vi "CameraVision_Demo_v02.vi"() -> (4 "图像时间戳":u32=16532020 format="%_32g")   [LabVIEW 2015]
uses:
  MVCAMSDK.dll
  <vilib>/Analysis/NI_AALBase.lvlib
panel:
  out "variance 2":dbl caption="方差2" format="%0.2f"
  out "光强图 2":u64[](graph)
  out "variance":dbl caption="方差" format="%0.2f"
  out "相机图像":T1(plugin-control)
  out "光强图":u64[](graph)
  in  "自定义分辨率设置":bool
  in  "ROI分辨率":T2
  in  "预设分辨率设置":bool
  in  "预设分辨率":T3(radio)
  out "帧速":u32
  out "帧间耗时\n单位：（0.1ms）":u32
  in  "相机枚举":T4(ring)
  in  "自动曝光模式":bool=TRUE caption="软触发"
  in  "手动曝光模式":bool caption="软触发"
  in  "曝光时间，单位微秒":dbl=11000.0 format="%#_6f"
  in  "硬触发模式":bool caption="软触发"
  in  "软触发模式":bool caption="软触发"
  in  "连续模式":bool caption="软触发"
  in  "软触发一帧":bool caption="软触发"
  in  "读取自定义数据":bool
  out "从相机中读出的字符串(32字节)":string
  in  "写入自定义数据":bool
  in  "要写入相机的字符串(32字节)":string
  in  "拍照":bool
  in  "相机参数":bool=TRUE
  in  "Stop":bool
  in  "激活预览":bool=TRUE
  out "Image":T1(plugin-control)
  # "写入自定义数据"
  # "相机原生分辨率设置"
  # "触发设置"
  # "曝光设置"
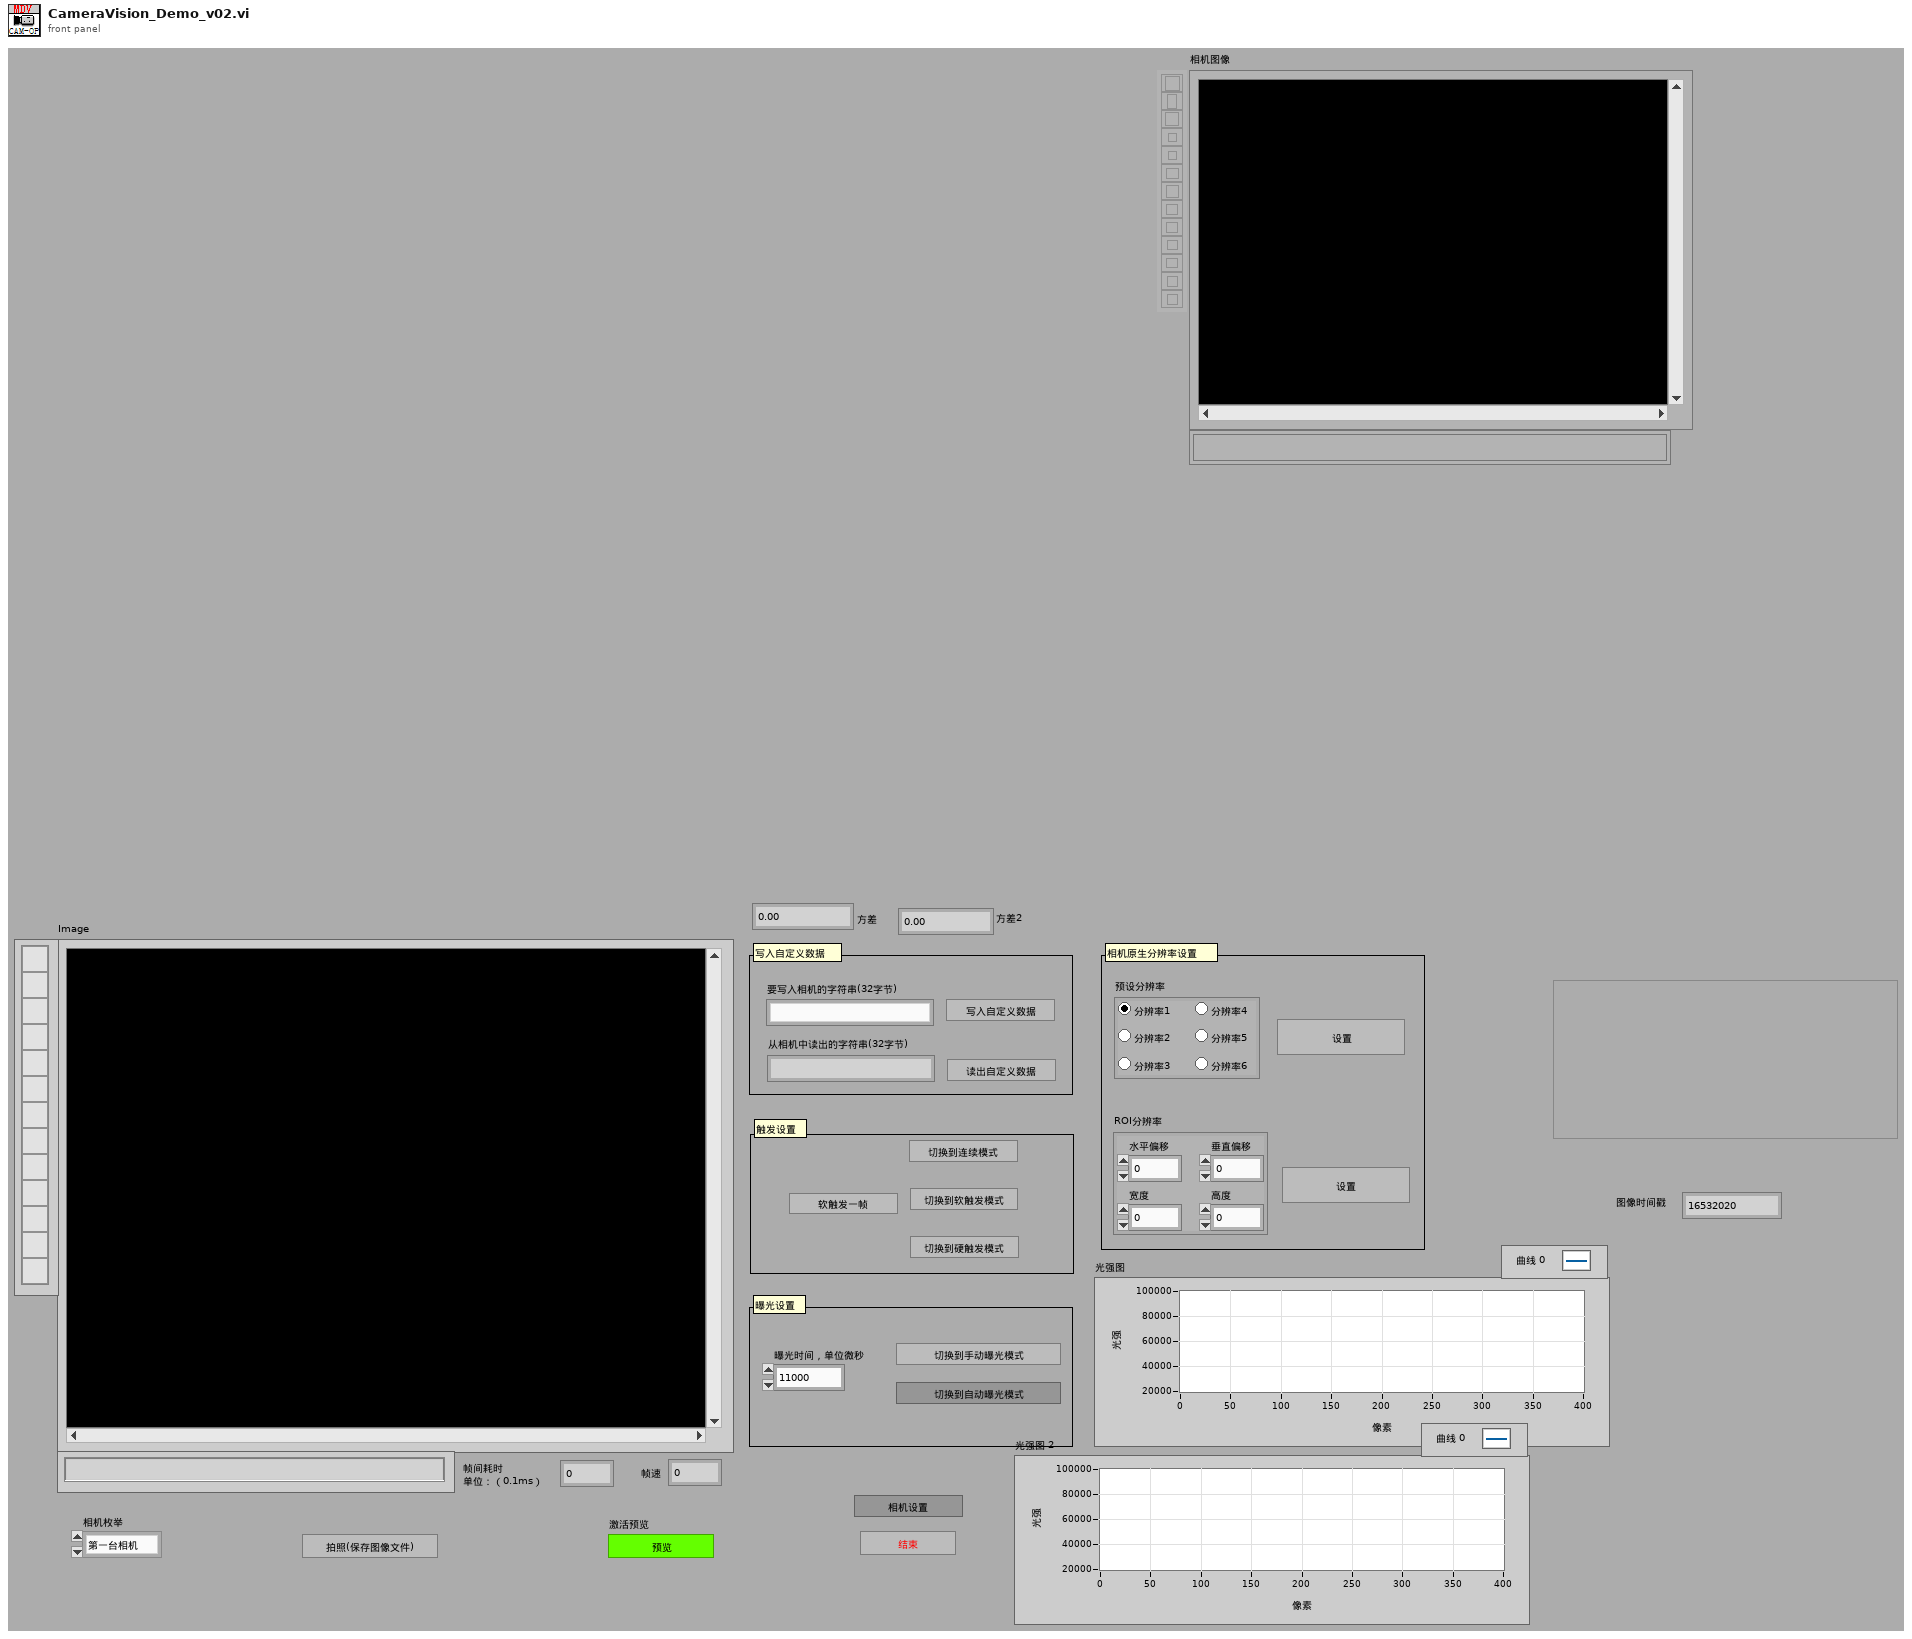
[diagram p1: front panel]
types:
  T1 = typedef "IMAQ Image.ctl" = refnum<image>
  T2 = cluster{"水平偏移":dbl, "垂直偏移":dbl, "宽度":dbl, "高度":dbl}
  T3 = enum32{"分辨率1", "分辨率2", "分辨率3", "分辨率4", "分辨率5", "分辨率6"}
  T4 = enum16{"第一台相机", "第二台相机", "第三台相机", "第四台相机", "第五台相机"}
  T5 = typedef "Image Type" = u32
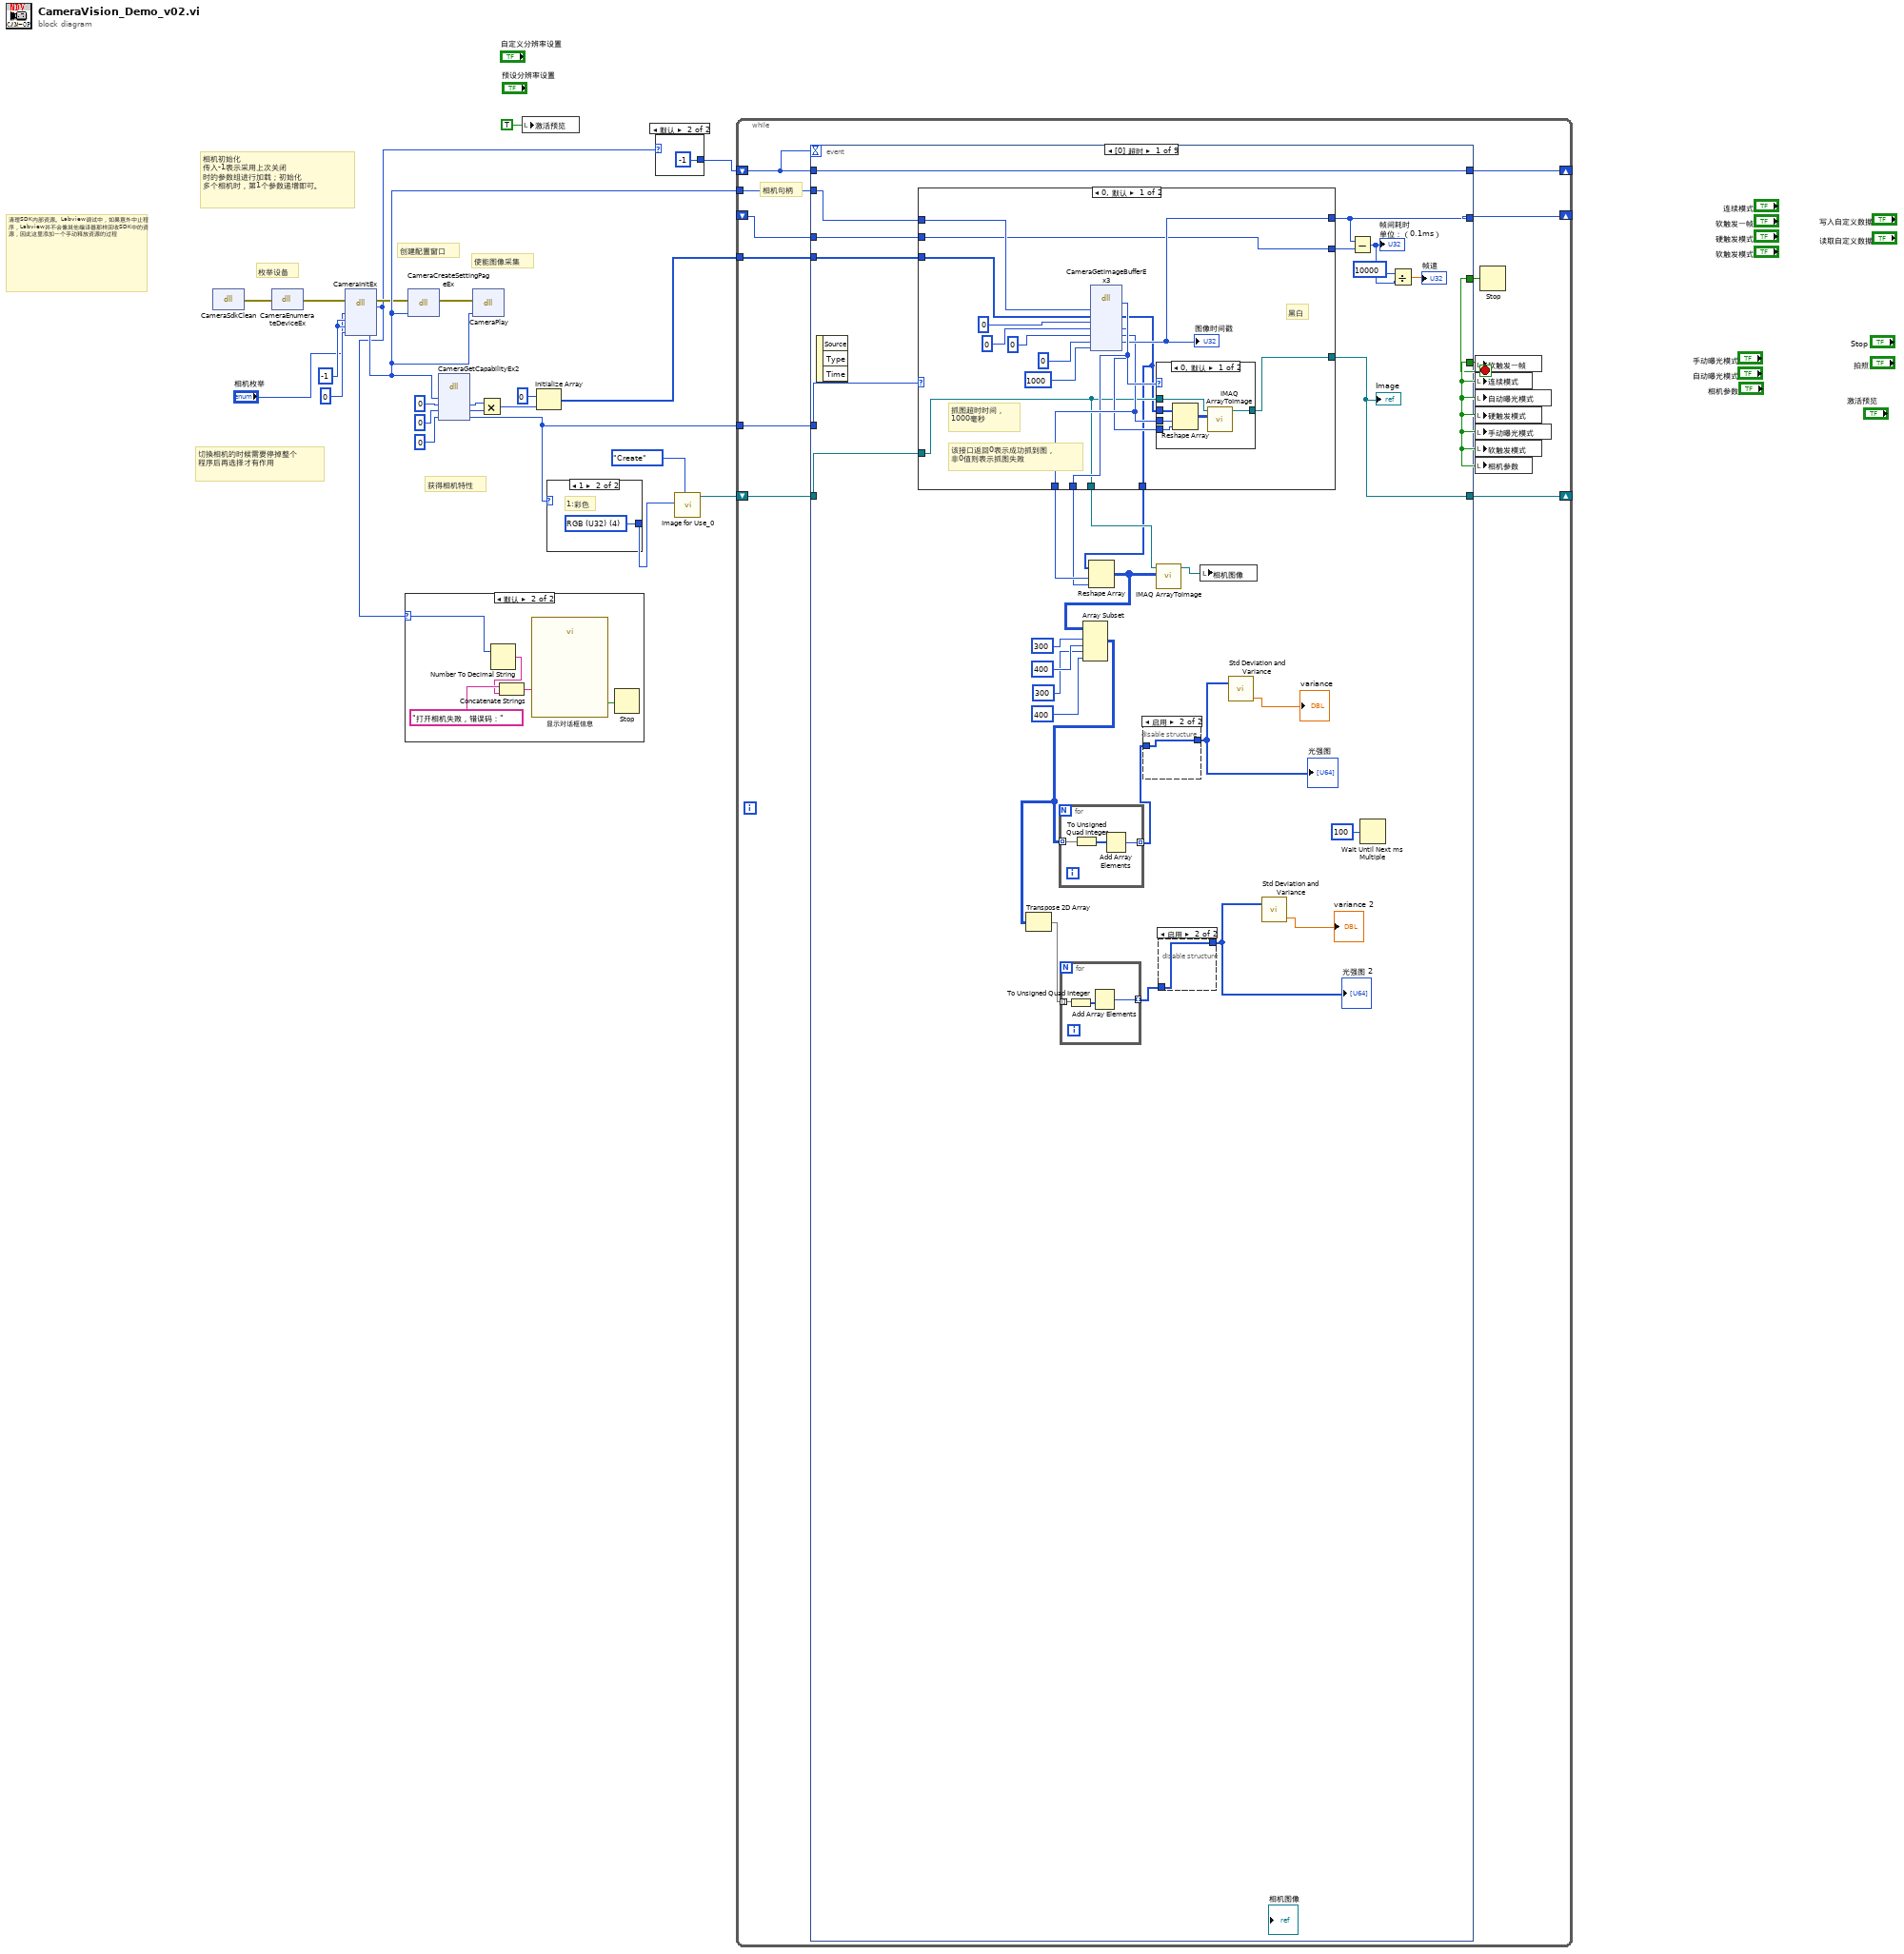
[diagram p0: block diagram]
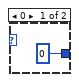
[diagram p2: hidden frame]
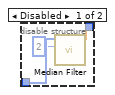
[diagram p4: hidden frame]
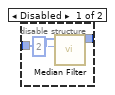
[diagram p5: hidden frame]
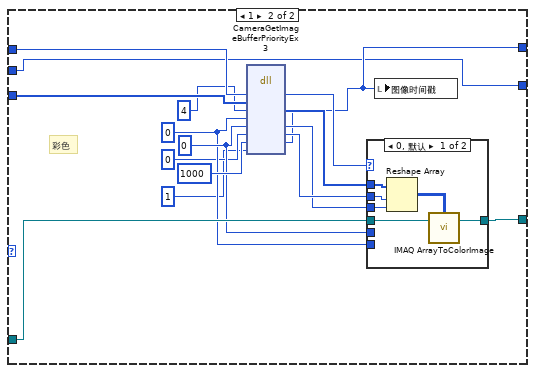
[diagram p7: hidden frame]
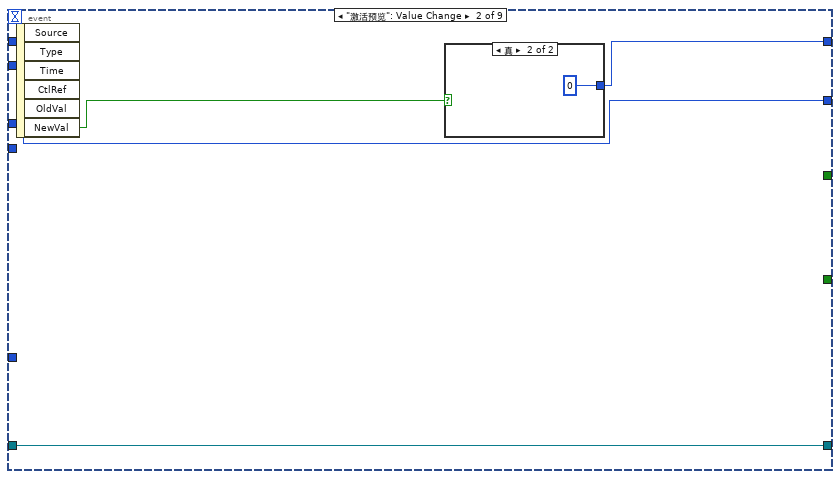
[diagram p9: hidden frame]
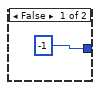
[diagram p10: hidden frame]
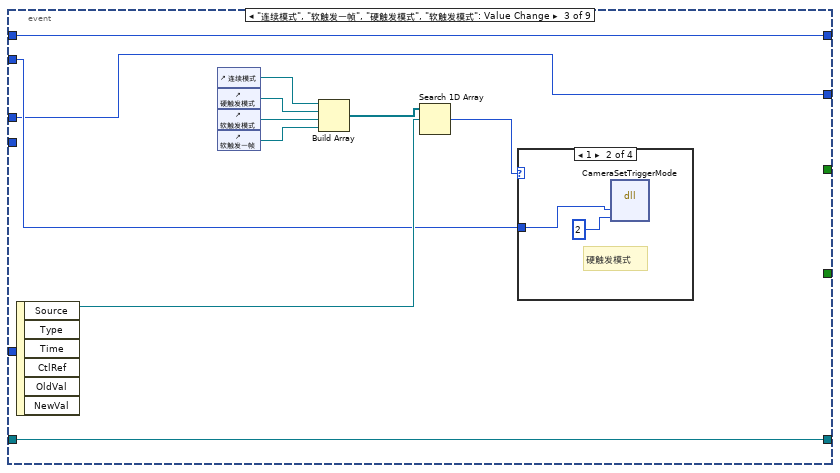
[diagram p11: hidden frame]
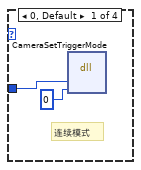
[diagram p12: hidden frame]
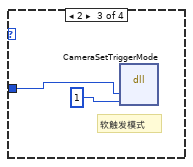
[diagram p13: hidden frame]
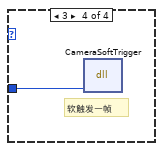
[diagram p14: hidden frame]
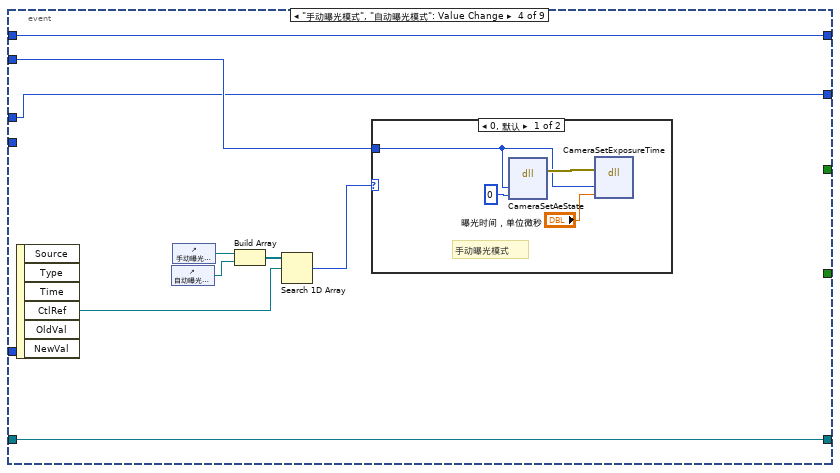
[diagram p15: hidden frame]
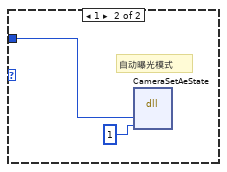
[diagram p16: hidden frame]
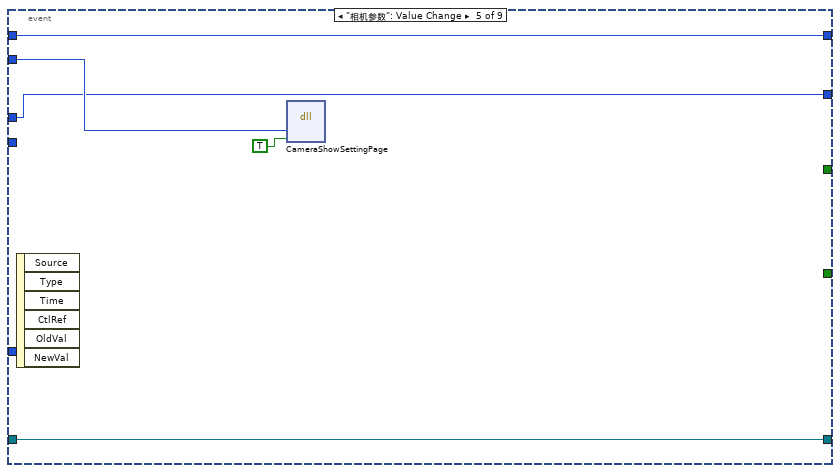
[diagram p17: hidden frame]
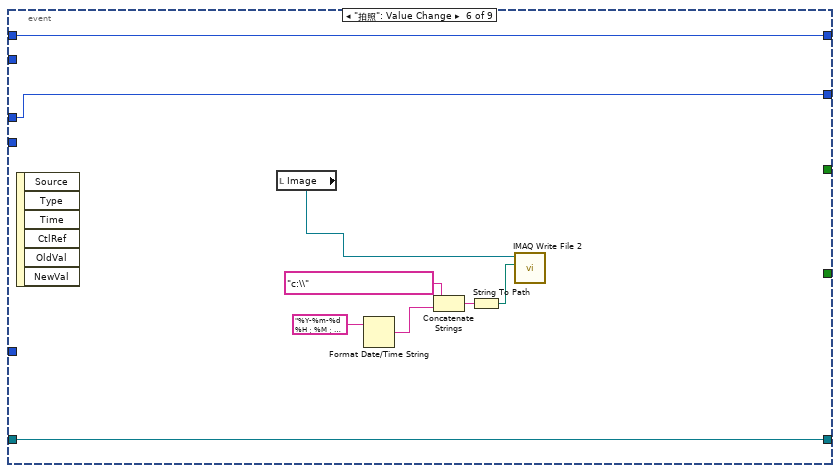
[diagram p18: hidden frame]
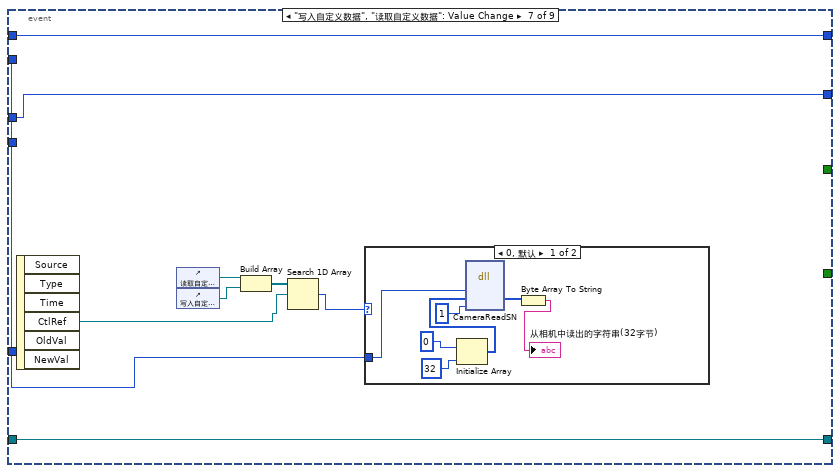
[diagram p19: hidden frame]
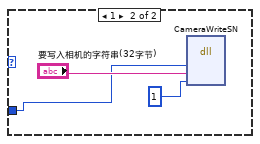
[diagram p20: hidden frame]
diagram:
  w20 = -1
  # "切换相机的时候需要停掉整个\n程序后再选择才有作用"
  # "清理SDK内部资源。Labview调试中，如果意外中止程序，Labview并不会像其他编译器那样回收SDK中的资源，因此这里添加一个手动释放资源的过程"
  # "使能图像采集"
  # "获得相机特性"
  # "创建配置窗口"
  # "相机初始化\n传入-1表示采用上次关闭\n时的参数组进行加载；初始化\n多个相机时，第1个参数递增即可。"
  # "枚举设备"
  n1 = dll-call lib="MVCAMSDK.dll" fn="CameraSdkClean"() -> (error out=w21:errorcluster)  [unwired: 4 in, 1 out]
  n2 = dll-call lib="MVCAMSDK.dll" fn="CameraEnumerateDeviceEx"(error in=w21) -> (error out=w18:errorcluster)  [unwired: 3 in, 1 out]
  n3 = dll-call lib="MVCAMSDK.dll" fn="CameraInitEx"(error in=w18, "相机索引值"="相机枚举", "参数加载方式"=w20, "要加载的参数组索引"=w20, "相机句柄"=0) -> (error out=w7:errorcluster, "返回类型"=w2:i32, "相机句柄"=w9:i32)  [unwired: 5 in, 1 out]
  n4 = case shown="默认" w2 {
    selector: w2 -> [_ w27]
    frame 0 {
    }
    frame Default {
      n5 = Number To Decimal String(number=w27) -> (decimal integer string=w24:string)  [unwired: 1 in]
      n6 = Concatenate Strings("打开相机失败，错误码：" ("字符串"), w24) -> (w26:string)
      n7 = call "显示对话框信息"("Message"=w26) -> ("结束"=w28:bool)  [unwired: 9 in, 1 out]
      n8 = Stop(stop? (T)=w28) -> ()
    }
  }
  n9 = dll-call lib="MVCAMSDK.dll" fn="CameraCreateSettingPageEx"(error in=w7, "相机句柄"=w9) -> (error out=w10:errorcluster)  [unwired: 4 in, 1 out]
  n10 = dll-call lib="MVCAMSDK.dll" fn="CameraGetCapabilityEx2"("相机句柄"=w9, "图像最大宽度"=0, "图像最大高度"=0, "是否是彩色相机(返回0:黑白;1:彩色)"=0) -> ("图像最大宽度"=w12:i32, "图像最大高度"=w11:i32, "是否是彩色相机(返回0:黑白;1:彩色)"=w6:i32)  [unwired: 5 in, 2 out]
  n11 = dll-call lib="MVCAMSDK.dll" fn="CameraPlay"(error in=w10, "相机句柄"=w9) -> ()  [unwired: 4 in, 2 out]
  n12 = Multiply(x=w12, y=w11) -> (x*y=w16:i32)
  n13 = local write "激活预览"(TRUE ("激活预览")) -> ()
  n14 = Initialize Array(0, w16) -> (w8:i32[])
  n15 = case shown="1" w6 {
    tunnel: [_ w29] -> w22
    frame 0, Default {
      # "0:黑白;"
    }
    frame 1 {
      w29 = T5 4 items=["Grayscale (U8)", "Grayscale (I16)", "Grayscale (SGL)", "Complex (CSG)", "RGB (U32)", "HSL (U32)", "RGB (U64)", "Grayscale (U16)"] ("Image Type")
      # "1:彩色"
    }
  }
  n16 = case shown="默认" w2 {
    tunnel: [0 -1] -> w1
    frame 0 {
    }
    frame Default {
    }
  }
  n17 = call "Image for Use_0.vi"("Command"=enum16{"Create", "Use", "Copy in", "Dispose"}."Create", "Image Type"=w22) -> ("Image out"=w5:T1)  [unwired: 8 in, 1 out]
  n18 = while {
    tunnel: w9 -> [w39]
    tunnel: w8 -> [w41]
    tunnel: w6 -> [w42]
    shift-right: [w38] -> _
    shift-left: w1 -> [w37]
    shift-right: [w35] -> _
    shift-left: w5 -> [w40]
    shift-right: [w34] -> _
    shift-left: _ -> [w33]
    stop <- w32 stop-if-true
    # "相机句柄"
    n19 = event shown="[0] 超时" {
      selector: _ -> [_ _ _ _ _ _ _ _ _]
      dyn-events: _ -> [_ _ _ _ _ _ _ _ _]
      timeout: w37 -> [_ _ _ _ _ _ _ _ _]
      tunnel: [_ _ _ _ _ _ _ _ TRUE] -> w32
      tunnel: w41 -> [w72 _ _ _ _ _ _ _ _]
      tunnel: w42 -> [w71 _ _ _ _ _ _ _ _]
      tunnel: w39 -> [w73 _ w141 w159 w174 _ w188 w211 w291]
      tunnel: w40 -> [w70 w134 w140 w158 w173 w178 w187 w213 w289]
      tunnel: [w69 w135 w142 w160 w175 w179 w189 w214 w292] -> w38
      tunnel: w37 -> [w69 _ w142 w160 w175 w179 w189 w214 w292]
      tunnel: [_ _ _ _ _ _ _ _ FALSE] -> w36
      tunnel: [w68 w134 w140 w158 w173 w178 w187 w213 w289] -> w35
      tunnel: [w65 w133 w139 w157 w172 w177 w186 w205 w288] -> w34
      tunnel: w33 -> [w67 w133 w139 w157 w172 w177 w186 w205 w288]
      event Timeout {
        n20 = event-data() -> ()  [unwired: 1 in, 3 out]
        n21 = case shown="0, 默认" w71 {
          tunnel: w72 -> [w102 w125]
          tunnel: w70 -> [w89 w124]
          tunnel: w73 -> [w94 w123]
          tunnel: [w95 w113] -> w68
          tunnel: [w93 w112] -> w65
          tunnel: w67 -> [w92 w111]
          tunnel: [w92 w111] -> w66
          tunnel: [w91 _] -> w59
          tunnel: [w90 _] -> w58
          tunnel: [w89 _] -> w57
          tunnel: [w88 _] -> w56
          frame 0, Default {
            # "黑白"
            # "该接口返回0表示成功抓到图，\n非0值则表示抓图失败"
            # "抓图超时时间，\n1000毫秒"
            n22 = dll-call lib="MVCAMSDK.dll" fn="CameraGetImageBufferEx3"("相机句柄"=w94, "图像数据缓冲区"=w102, "图像输出格式(0:8位灰度;1:24位彩色;2:32位彩色，3：BGR24彩色 4：BGRA32位彩色)"=0, "图像宽度"=0, "图像高度"=0, "时间戳(单位为100微秒)"=0, "抓图超时时间(毫秒)"=1000) -> ("返回类型"=w97:i32, "图像数据缓冲区"=w88:u8[], "图像宽度"=w90:i32, "图像高度"=w91:i32, "时间戳(单位为100微秒)"=w93:u32)  [unwired: 6 in, 2 out]
            "图像时间戳" <- w93
            n23 = case shown="0, 默认" w97 {
              tunnel: w88 -> [w108 _]
              tunnel: w89 -> [w105 w109]
              tunnel: w91 -> [w107 _]
              tunnel: w90 -> [w106 _]
              tunnel: [w103 w109] -> w95
              frame 0, Default {
                n24 = Reshape Array(w108, w107, w106) -> (w104:u8[][])
                n25 = call "IMAQ ArrayToImage"("Image Pixels (U8)"=w104, "Image"=w105) -> ("Image Out"=w103:T1)  [unwired: 8 in, 1 out]
              }
              frame -12 {
              }
            }
          }
          frame 1 {
            w115 = 0
            w116 = 0
            # "彩色"
            n26 = dll-call lib="MVCAMSDK.dll" fn="CameraGetImageBufferPriorityEx3"("相机句柄"=w123, "图像数据缓冲区"=w125, "图像输出格式(0:8位灰度;1:24位彩色;2:32位彩色)"=4, "图像宽度"=w115, "图像高度"=w116, "时间戳（单位为100微秒）"=0, "抓图超时时间(毫秒)"=1000, "取图优先级(0: 取最旧   1:取最新)"=1) -> ("返回类型"=w117:i32, "图像数据缓冲区"=w120:u32[], "图像宽度"=w118:i32, "图像高度"=w119:i32, "时间戳（单位为100微秒）"=w112:u32)  [unwired: 7 in, 2 out]
            n27 = case shown="0, 默认" w117 {
              tunnel: w120 -> [w130 _]
              tunnel: w124 -> [w129 w132]
              tunnel: w119 -> [w128 _]
              tunnel: w118 -> [w127 _]
              tunnel: w116 -> [_ _]
              tunnel: w115 -> [_ _]
              tunnel: [w126 w132] -> w113
              frame 0, Default {
                n28 = Reshape Array(w130, w128, w127) -> (w131:u32[][])
                n29 = call "IMAQ ArrayToColorImage"("Image Pixels (U32)"=w131, "Image"=w129) -> ("Image Out"=w126:T1)  [unwired: 3 in, 1 out]
              }
              frame -12 {
              }
            }
            n30 = local write "图像时间戳"(w112) -> ()
          }
        }
        "Image" <- w68
        n31 = Reshape Array(w56, w59, w58) -> (w44:u8[][])
        n32 = Array Subset(array=w44, index (row)=300 ("索引"), length (row)=400 ("长度"), index (col)=300 ("长度"), length (col)=400 ("索引")) -> (w43:u8[][])
        n33 = Transpose 2D Array(2D array=w43) -> (transposed array=w51:u8[][])
        n34 = for {
          tunnel: w43 -> [w82] mode=indexing
          tunnel: [w83] -> w54 mode=indexing
          n35 = To Unsigned Quad Integer(1:w82) -> (0:w81:u64[])
          n36 = Add Array Elements(numeric array=w81) -> (sum=w83:u64)
        }
        n37 = for {
          tunnel: w51 -> [w75] mode=indexing
          tunnel: [w76] -> w52 mode=indexing
          n38 = To Unsigned Quad Integer(1:w75) -> (0:w74:u64[])
          n39 = Add Array Elements(numeric array=w74) -> (sum=w76:u64)
        }
        n40 = disable-structure shown="启用" {
          disable-tunnel: w54 -> [w86 w87]
          disable-tunnel: [w84 w87] -> w50
          frame Disabled {
            n41 = call <vilib>:"Median Filter.vi"("left rank"=2, "X"=w86) -> ("Filtered X"=w84:dbl[])  [unwired: 8 in, 1 out]
          }
          frame Enabled {
          }
        }
        "光强图" <- w50
        n42 = call "IMAQ ArrayToImage"("Image Pixels (U8)"=w44, "Image"=w57) -> ("Image Out"=w60:T1)  [unwired: 8 in, 1 out]
        n43 = disable-structure shown="启用" {
          disable-tunnel: w52 -> [w79 w80]
          disable-tunnel: [w77 w80] -> w49
          frame Disabled {
            n44 = call <vilib>:"Median Filter.vi"("left rank"=2, "X"=w79) -> ("Filtered X"=w77:dbl[])  [unwired: 8 in, 1 out]
          }
          frame Enabled {
          }
        }
        "光强图 2" <- w49
        n45 = local write "相机图像"(w60) -> ()
        n46 = call <vilib>:"Std Deviation and Variance.vi"("X"=w50) -> ("variance"=→"variance":dbl)  [unwired: 1 in, 2 out]
        n47 = call <vilib>:"Std Deviation and Variance.vi"("X"=w49) -> ("variance"=→"variance 2":dbl)  [unwired: 1 in, 2 out]
        n48 = Subtract(x=w65, y=w66) -> (x-y=w64:u32)
        "帧间耗时\n单位：（0.1ms）" <- w64
        n49 = Wait Until Next ms Multiple(millisecond multiple=u32 100 ("毫秒倍数")) -> ()  [unwired: 1 out]
        n50 = Divide(x=u32 10000 ("帧间耗时"), y=w64) -> (x/y=→"帧速":dbl)
      }
      event "激活预览": Value Change {
        n51 = event-data() -> ("NewVal"=w136:bool)  [unwired: 1 in, 5 out]
        n52 = case shown="真" w136 {
          tunnel: [-1 0] -> w135
          frame False {
          }
          frame True {
          }
        }
      }
      event "连续模式", "软触发一帧", "硬触发模式", "软触发模式": Value Change {
        n53 = event-data() -> ("CtlRef"=w144:refnum<vi>)  [unwired: 1 in, 5 out]
        n54 = control-ref of="连续模式"() -> (w146:refnum<vi>)
        n55 = control-ref of="硬触发模式"() -> (w147:refnum<vi>)
        n56 = control-ref of="软触发模式"() -> (w148:refnum<vi>)
        n57 = control-ref of="软触发一帧"() -> (w149:refnum<vi>)
        n58 = Build Array ("创建数组")(w146, w147, w148, w149) -> (w145:refnum<vi>[])
        n59 = Search 1D Array(1D array=w145, element=w144) -> (index of element=w143:i32)  [unwired: 1 in]
        n60 = case shown="1" w143 {
          tunnel: w141 -> [w150 w152 w154 w156]
          frame 0, Default {
            # "连续模式"
            n61 = dll-call lib="MVCAMSDK.dll" fn="CameraSetTriggerMode"("相机句柄"=w150, "模式"=0) -> ()  [unwired: 6 in, 2 out]
          }
          frame 1 {
            # "硬触发模式"
            n62 = dll-call lib="MVCAMSDK.dll" fn="CameraSetTriggerMode"("相机句柄"=w152, "模式"=2) -> ()  [unwired: 6 in, 2 out]
          }
          frame 2 {
            # "软触发模式"
            n63 = dll-call lib="MVCAMSDK.dll" fn="CameraSetTriggerMode"("相机句柄"=w154, "模式"=1) -> ()  [unwired: 6 in, 2 out]
          }
          frame 3 {
            # "软触发一帧"
            n64 = dll-call lib="MVCAMSDK.dll" fn="CameraSoftTrigger"("相机句柄"=w156) -> ()  [unwired: 5 in, 2 out]
          }
        }
      }
      event "手动曝光模式", "自动曝光模式": Value Change {
        n65 = event-data() -> ("CtlRef"=w163:refnum<vi>)  [unwired: 1 in, 5 out]
        n66 = control-ref of="自动曝光模式"() -> (w161:refnum<vi>)
        n67 = control-ref of="手动曝光模式"() -> (w164:refnum<vi>)
        n68 = Build Array ("创建数组")(w164, w161) -> (w165:refnum<vi>[])
        n69 = Search 1D Array(1D array=w165, element=w163) -> (index of element=w162:i32)  [unwired: 1 in]
        n70 = case shown="0, 默认" w162 {
          tunnel: w159 -> [w166 w170]
          frame 0, Default {
            # "手动曝光模式"
            n71 = dll-call lib="MVCAMSDK.dll" fn="CameraSetAeState"("相机句柄"=w166, "曝光模式(0手动，1自动)"=0) -> (error out=w169:errorcluster)  [unwired: 6 in, 1 out]
            n72 = dll-call lib="MVCAMSDK.dll" fn="CameraSetExposureTime"(error in=w169, "相机句柄"=w166, "曝光时间，单位微秒"="曝光时间，单位微秒") -> ()  [unwired: 5 in, 2 out]
          }
          frame 1 {
            # "自动曝光模式"
            n73 = dll-call lib="MVCAMSDK.dll" fn="CameraSetAeState"("相机句柄"=w170, "曝光模式(0手动，1自动)"=1) -> ()  [unwired: 6 in, 2 out]
          }
        }
      }
      event "相机参数": Value Change {
        n74 = event-data() -> ()  [unwired: 1 in, 6 out]
        n75 = dll-call lib="MVCAMSDK.dll" fn="CameraShowSettingPage"("相机句柄"=w174, "状态"=TRUE) -> ()  [unwired: 6 in, 2 out]
      }
      event "拍照": Value Change {
        n76 = event-data() -> ()  [unwired: 1 in, 6 out]
        n77 = local read "Image"() -> (w180:T1)
        n78 = Format Date/Time String(time format string (%c)="%Y-%m-%d %H：%M：%S.bmp ") -> (date/time string=w184:string)  [unwired: 2 in]
        n79 = Concatenate Strings("c:\\", w184) -> (w181:string)
        n80 = String To Path(string=w181) -> (path=w183:path)
        n81 = call-poly "IMAQ Write File 2"("File Path"=w183, "Image"=w180) -> ()  [unwired: 8 in, 2 out]
      }
      event "写入自定义数据", "读取自定义数据": Value Change {
        n82 = event-data() -> ("CtlRef"=w191:refnum<vi>)  [unwired: 1 in, 5 out]
        n83 = control-ref of="读取自定义数据"() -> (w193:refnum<vi>)
        n84 = control-ref of="写入自定义数据"() -> (w192:refnum<vi>)
        n85 = Build Array ("创建数组")(w193, w192) -> (w194:refnum<vi>[])
        n86 = Search 1D Array(1D array=w194, element=w191) -> (index of element=w190:i32)  [unwired: 1 in]
        n87 = case shown="0, 默认" w190 {
          tunnel: w188 -> [w195 w202]
          frame 0, Default {
            n88 = Initialize Array(0, 32) -> (w199:i32[])
            n89 = dll-call lib="MVCAMSDK.dll" fn="CameraReadSN"("相机句柄"=w195, "序列号"=w199, "序列号级别，[0,1,2],0级为只读，1,2级可写"=1) -> ("序列号"=w197:u8[])  [unwired: 6 in, 2 out]
            n90 = Byte Array To String(unsigned byte array=w197) -> (string=→"从相机中读出的字符串(32字节)":string)
          }
          frame 1 {
            n91 = dll-call lib="MVCAMSDK.dll" fn="CameraWriteSN"("相机句柄"=w202, "序列号(固定为32个字节)"="要写入相机的字符串(32字节)", "序列号级别，[0,1,2]对应3级序列号，其中0级为只读，1,2级可写"=1) -> ()  [unwired: 7 in, 2 out]
          }
        }
      }
      event "预设分辨率设置", "自定义分辨率设置": Value Change {
        n92 = event-data() -> ("CtlRef"=w207:refnum<vi>)  [unwired: 1 in, 5 out]
        n93 = control-ref of="预设分辨率设置"() -> (w209:refnum<vi>)
        n94 = control-ref of="自定义分辨率设置"() -> (w208:refnum<vi>)
        n95 = Build Array ("创建数组")(w209, w208) -> (w210:refnum<vi>[])
        n96 = Search 1D Array(1D array=w210, element=w207) -> (index of element=w206:i32)  [unwired: 1 in]
        n97 = case shown="1" w206 {
          tunnel: "预设分辨率" -> [w216 _]
          tunnel: w211 -> [w215 w277]
          frame 0, Default {
            n98 = case shown="\"分辨率2\"" w216 {
              tunnel: w215 -> [w217 w236 w237 w247 w257 w267]
              frame "分辨率1", Default {
                n99 = dll-call lib="MVCAMSDK.dll" fn="CameraSetImageResolutionEx"("相机句柄"=w217, "预设分辨率索引"=0, "Mode"=0, "ModeSize"=u32 0, "x"=0, "y"=u32 0 ("ModeSize"), "width"=0, "height"=0, "ZoomWidth"=0, "ZoomHeight"=0) -> ()  [unwired: 14 in, 2 out]
              }
              frame "分辨率2" {
                n100 = dll-call lib="MVCAMSDK.dll" fn="CameraSetImageResolutionEx"("相机句柄"=w236, "预设分辨率索引"=1, "Mode"=0, "ModeSize"=u32 0, "x"=0, "y"=u32 0 ("ModeSize"), "width"=0, "height"=0, "ZoomWidth"=0, "ZoomHeight"=0) -> ()  [unwired: 14 in, 2 out]
              }
              frame "分辨率3" {
                n101 = dll-call lib="MVCAMSDK.dll" fn="CameraSetImageResolutionEx"("相机句柄"=w237, "预设分辨率索引"=2, "Mode"=0, "ModeSize"=u32 0, "x"=0, "y"=u32 0 ("ModeSize"), "width"=0, "height"=0, "ZoomWidth"=0, "ZoomHeight"=0) -> ()  [unwired: 14 in, 2 out]
              }
              frame "分辨率4" {
                n102 = dll-call lib="MVCAMSDK.dll" fn="CameraSetImageResolutionEx"("相机句柄"=w247, "预设分辨率索引"=3, "Mode"=0, "ModeSize"=u32 0, "x"=0, "y"=u32 0 ("ModeSize"), "width"=0, "height"=0, "ZoomWidth"=0, "ZoomHeight"=0) -> ()  [unwired: 14 in, 2 out]
              }
              frame "分辨率5" {
                n103 = dll-call lib="MVCAMSDK.dll" fn="CameraSetImageResolutionEx"("相机句柄"=w257, "预设分辨率索引"=4, "Mode"=0, "ModeSize"=u32 0, "x"=0, "y"=u32 0 ("ModeSize"), "width"=0, "height"=0, "ZoomWidth"=0, "ZoomHeight"=0) -> ()  [unwired: 14 in, 2 out]
              }
              frame "分辨率6" {
                n104 = dll-call lib="MVCAMSDK.dll" fn="CameraSetImageResolutionEx"("相机句柄"=w267, "预设分辨率索引"=5, "Mode"=0, "ModeSize"=u32 0, "x"=0, "y"=u32 0 ("ModeSize"), "width"=0, "height"=0, "ZoomWidth"=0, "ZoomHeight"=0) -> ()  [unwired: 14 in, 2 out]
              }
            }
          }
          frame 1 {
            n105 = Unbundle("ROI分辨率") -> ("水平偏移"=w279:dbl, "垂直偏移"=w280:dbl, "宽度"=w281:dbl, "高度"=w282:dbl)
            n106 = dll-call lib="MVCAMSDK.dll" fn="CameraSetImageResolutionEx"("相机句柄"=w277, "预设分辨率索引"=255, "Mode"=0, "ModeSize"=u32 0, "x"=w279, "y"=w280, "width"=w281, "height"=w282, "ZoomWidth"=0, "ZoomHeight"=u32 0 ("ModeSize")) -> ()  [unwired: 14 in, 2 out]
          }
        }
      }
      event "Stop": Value Change {
        # "反初始化相机"
        n107 = event-data() -> ()  [unwired: 1 in, 6 out]
        n108 = dll-call lib="MVCAMSDK.dll" fn="CameraUnInit"("相机句柄"=w291) -> ()  [unwired: 5 in, 2 out]
      }
    }
    n109 = local write "软触发一帧"(w36) -> ()
    n110 = local write "连续模式"(w36) -> ()
    n111 = local write "自动曝光模式"(w36) -> ()
    n112 = local write "硬触发模式"(w36) -> ()
    n113 = local write "手动曝光模式"(w36) -> ()
    n114 = local write "软触发模式"(w36) -> ()
    n115 = local write "相机参数"(w36) -> ()
    n116 = Stop(stop? (T)=w32) -> ()
  }
